vi "requestSlitWidth.vi"(8 "error in (no error)":errorcluster, 10 "SlitType":T2, 11 "MonoClientCommunicator in":refnum<class "MonoClientCommunicator.lvclass">) -> (0 "error out":errorcluster, 2 "slitWidth":T1, 3 "MonoClientCommunicator out":refnum<class "MonoClientCommunicator.lvclass">)   [LabVIEW 2016, in "MonoClientCommunicator.lvclass"]
uses:
  MonoClientCommunicator.lvclass
  Typedefs/SlitType.ctl
  Typedefs/slitWidth.ctl
  Typedefs/MonoCommand.ctl
  Typedefs/publishers.ctl
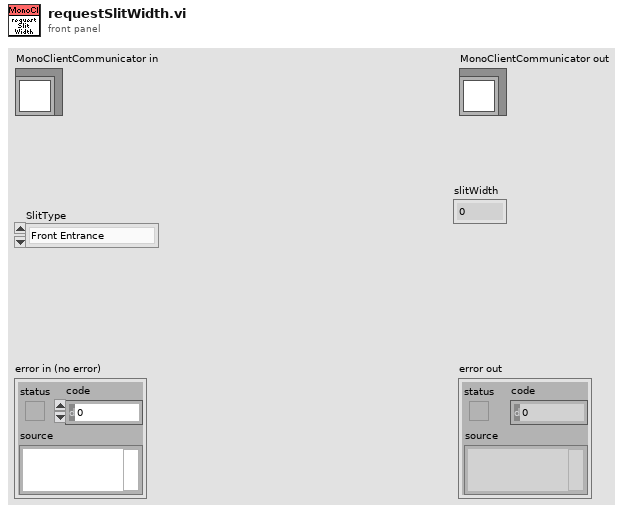
[diagram p1: front panel]
types:
  T1 = typedef "slitWidth.ctl" = dbl
  T2 = typedef "SlitType.ctl" = enum16{"Front Entrance", "Side Entrance", "Front Exit", "Side Exit", "First Intermediate", "Second Intermediate"}
  T3 = typedef "publishers.ctl" = enum16{"Wavelength", "Grating", "FrontEntranceSlitPosition", "FrontExitSlitPosition", "SoftwareStatus", "MonochromatorId", "Ack"}
  T4 = typedef "MonoCommand.ctl" = enum16{"getGrating", "getFrontEntranceSlitPosition", "getFrontExitSlitPosition", "getWavelength", "setWavelength", "setGrating", "setFrontEntranceSlitPosition", "setFrontExitSlitPosition", "calibrateWavelength", "getStatus", "Unknown", "reset"}
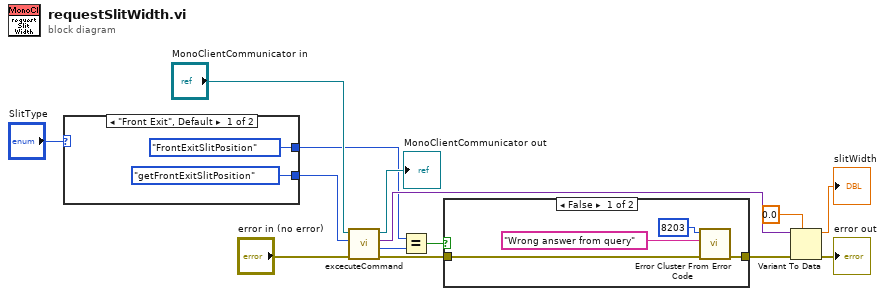
[diagram p0: block diagram]
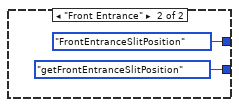
[diagram p3: hidden frame]
diagram:
  n1 = case shown="\"Front Exit\", Default" "SlitType" {
    tunnel: [MonoCommand."getFrontExitSlitPosition" ("MonoCommand") MonoCommand."getFrontEntranceSlitPosition" ("MonoCommand")] -> w2
    tunnel: [publishers."FrontExitSlitPosition" ("parameter") publishers."FrontEntranceSlitPosition" ("parameter")] -> w1
    frame "Front Exit", Default {
    }
    frame "Front Entrance" {
    }
  }
  n2 = call "excecuteCommand.vi"("error in (no error)"="error in (no error)", "MonoCommand"=w2, "MonoClientCommunicator in"="MonoClientCommunicator in") -> ("error out"=w9:errorcluster, "parameter"=w4:T3, "value"=w8:variant, "MonoClientCommunicator out"=→"MonoClientCommunicator out":refnum<class "MonoClientCommunicator.lvclass">)  [unwired: 5 in]
  n3 = Equal?(x=w1, y=w4) -> (x = y?=w3:bool)
  n4 = case shown="False" w3 {
    tunnel: w9 -> [w20 w23]
    tunnel: [w19 w23] -> w10
    frame False {
      n5 = call <vilib>:"Error Cluster From Error Code.vi"("error in (no error)"=w20, "error message (\"\")"="Wrong answer from query" ("error message (\"\")"), "error code (0)"=8203) -> ("error out"=w19:errorcluster)  [unwired: 6 in]
    }
    frame True {
    }
  }
  n6 = Variant To Data(error in=w10, type=T1 0.0 ("position"), Variant=w8) -> (data=→"slitWidth":T1, error out=→"error out":errorcluster)
